vi "Camera Light.vi"(2 "Error In":errorcluster, 3 "input":dbl=250.0) -> (0 "Error Out":errorcluster)   [LabVIEW 2016]
doc: "This example demonstrates how to configure the SPI master and do a data loopback test using a LINX device."
uses:
  <vilib>/MakerHub/LINX/Private/Type Defs/Peripherals/SPI/SPI Configuration.ctl
  <vilib>/MakerHub/LINX/Private/Type Defs/Peripherals/SPI/SPI Bit Order.ctl
  <vilib>/MakerHub/LINX/Private/Type Defs/Peripherals/SPI/SPI Mode.ctl
  <vilib>/MakerHub/LINX/Public/Peripherals/SPI/SPI CS Config.ctl
  <vilib>/MakerHub/LINX/Private/Type Defs/Peripherals/SPI/SPI CS Logic Level.ctl
  <vilib>/MakerHub/LINX/Public/Peripherals/SPI/SPI Write Read 1 Frame.vi
  <vilib>/MakerHub/LINX/Public/Peripherals/SPI/SPI Write Read N Frames.vi
  <vilib>/MakerHub/LINX/Private/Local IO/LinxSpiWriteRead.vi
  <vilib>/MakerHub/LINX/Public/Utilities/Check Channel.vi
  <vilib>/MakerHub/LINX/Public/Utilities/Open Serial.vi
  <vilib>/MakerHub/LINX/Private/Utilties/Generate Error.vi
  <vilib>/MakerHub/LINX/LMH-LINX.lvlib
panel:
  in  "Data":u8[](array[numeric])=[24, 3]
  in  "Serial Port":refnum<visa-resource-name>="COM4"
  out "Read Data 2":u8[](array[numeric])
  out "Read Data":u8[](array[numeric])
  in  "CS Configuration":T1={"CS Channel"=10, "CS Logic Level"=enum."Active Low"}
  out "Actual Clock Frequency":u32
  in  "SPI Configuration":T3={"Clock Frequency"=1000000, "Bit Order"=enum."MSb First", "SPI Mode"=enum."Mode 1"}
  # "SPI Loop Back Example\n\nThis example demonstrates how to configure the SPI master and write one frame of SPI data.\n\nInstructions\n0. Connect (short) the SPI MOSI and MOSI pins.\n1. Select the COM Port associated with the LINX Device.\n2. Select the SPI Configuration.\n3. Select the CS Configuration.\n4. Click the Run Arrow.\n5. Enter some data in the Write Data control.  Notice the output on the Read Data indicator."
  # "Designer : Chin-Chia Kuo"
  # "INTT"
  # "LINX Device Settings"
  # "SPI Master Settings"
  # "SPI Write / Read Configruation"
  # "chip pick up tool 210"
  # "kapton tape : 50"
  # "sensor 15"
  # "please setting from 0 to 255"
  # "Recommend value \nSensor : 15\nDrill hole : 250"
  # "SPI Master Settings\n1. Set the target SPI clock frequency.  \n   The possible frequencies varies by device and the actual frequency used is returned.\n2. The bit order determines the order that the individual bits in each byte are shifted out.\n3. SPI Mode determines the clock polarity and phase. (View context help on the SPI Configure VI for more information)"
  # "SPI Write / Read Configuration\n1. Select the CS (chip select) DO channel.  The channel is automatically set as an output.\n2. Select the logic level for the CS pin.\n3. CS is automatically toggled each when the SPI Write / Read VI executes."
  # "SPI Write / Read Frame\n1. A 'frame' is one SPI transaction.  It starts when CS goes active and ends when CS returns to the idle state.\n2. A frame can be an arbitrary number for bytes in lenght.\n3. When using the SPI Write / Read VI in 1 Frame mode all data bytes are sent in a single frame.  For example if the data array contains 4 bytes all 4 bytes are sent as a single frame.\n4. When using the SPI Write / Read in N Frames mode the data bytes are divided into multiple frames.  \n    For example if the data array contains 4 bytes and the frame size is set to 2 the SPI Write / Read VI will send 2 frames of 2 bytes each.\n    The number of data bytes must be evenly divisble by the frame size."
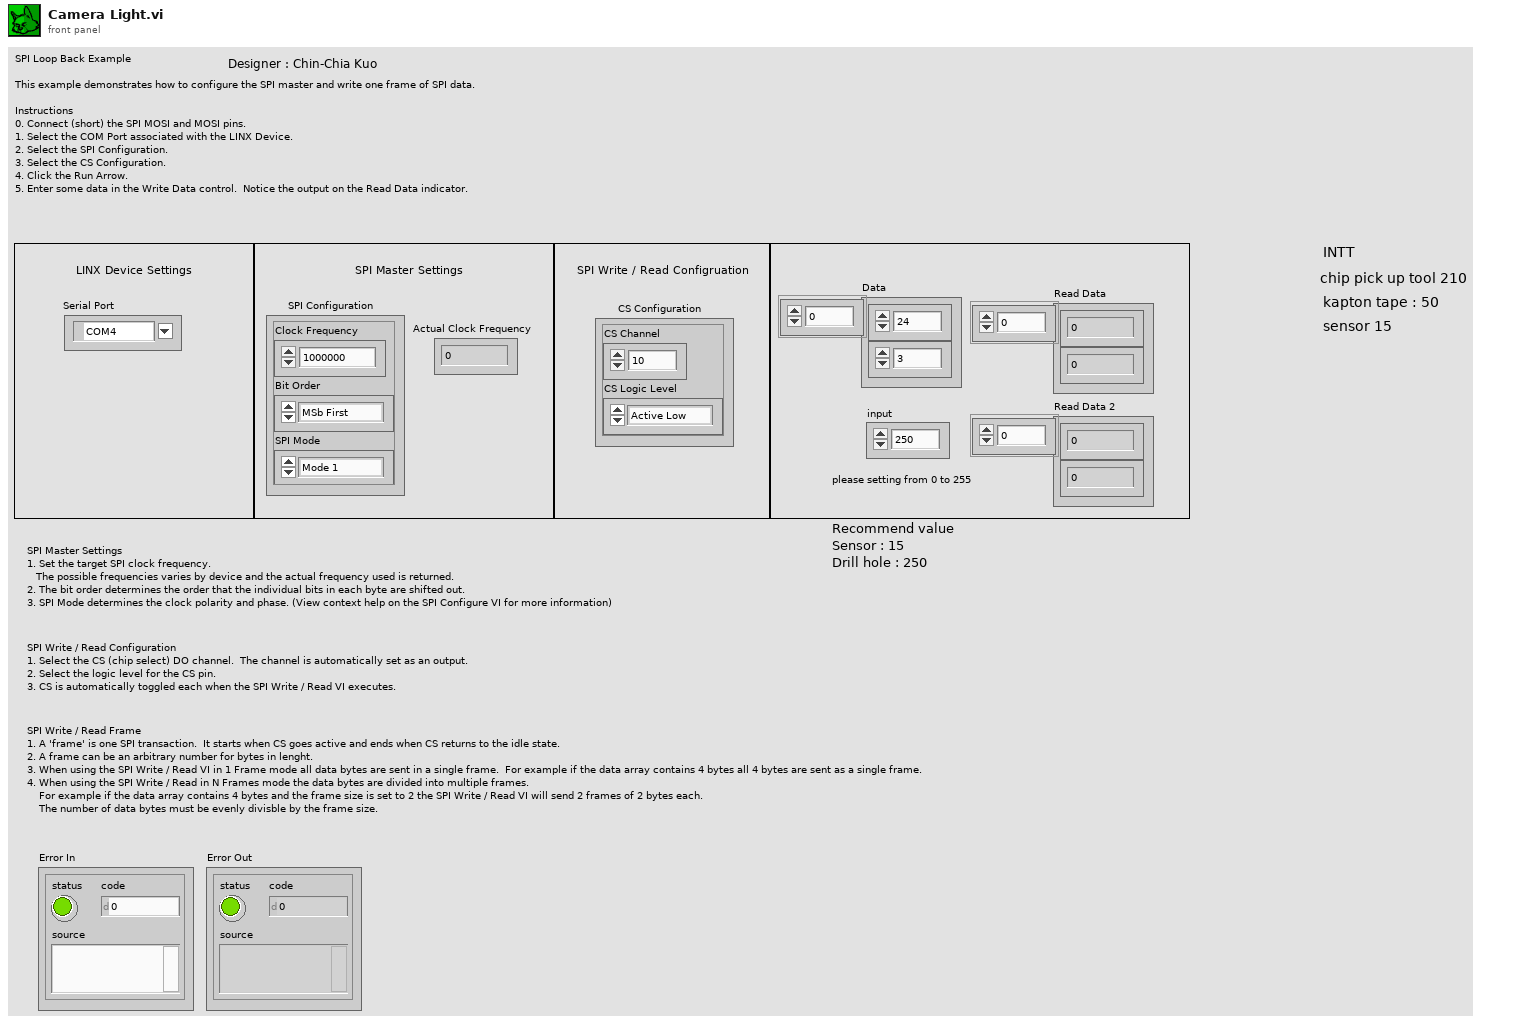
[diagram p1: front panel]
types:
  T1 = typedef "LMH-LINX.lvlib/SPI CS Config.ctl" = cluster{"CS Channel":u8, "CS Logic Level":T2}
  T2 = typedef "LMH-LINX.lvlib/SPI CS Logic Level.ctl" = enum8{"Active Low", "Active High"}
  T3 = typedef "LMH-LINX.lvlib/SPI Configuration.ctl" = cluster{"Clock Frequency":u32, "Bit Order":T4, "SPI Mode":T5}
  T4 = typedef "LMH-LINX.lvlib/SPI Bit Order.ctl" = enum8{"LSb First", "MSb First"}
  T5 = typedef "LMH-LINX.lvlib/SPI Mode.ctl" = enum8{"Mode 0", "Mode 1", "Mode 2", "Mode 3"}
  T6 = typedef "LMH-LINX.lvlib/LINX Ref.ctl" = cluster{"IO":T7, "Interface":T8, "LINX Device Config":T9}
  T7 = typedef "LMH-LINX.lvlib/Platform.ctl" = enum16{"Remote", "Local"}
  T8 = typedef "LMH-LINX.lvlib/Interface.ctl" = enum16{"Serial", "TCP"}
  T9 = typedef "LMH-LINX.lvlib/Device.lvlib/LINX Device Config.ctl" = cluster{"Interface":T8, "COM Port":refnum<visa-resource-name>, "TCP Configuration":T10, "Device Family":u8, "Device ID":u8, "Device Name":string, "TCP Ref":refnum<k5>, "Channels":T11}
  T10 = typedef "LMH-LINX.lvlib/Device.lvlib/TCP Config.ctl" = cluster{"IP Address":string, "Port":u16}
  T11 = typedef "LMH-LINX.lvlib/Channels.ctl" = cluster{"DI":u8[], "DO":u8[], "AI":u8[], "AO":u8[], "PWM":u8[], "QE":u8[], "UART":u8[], "I2C 2":u8[], "SPI":u8[], "CAN":u8[], "Servo":u8[], "AI Ref (V)":dbl, "AI Resolution (Bits)":u8, "AO Ref (V)":dbl, "AO Resolution (Bits)":u8}
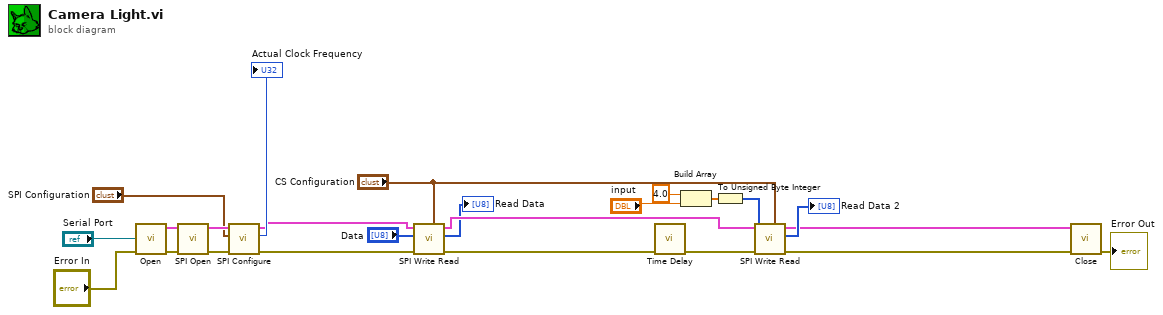
[diagram p0: block diagram]
diagram:
  n1 = call-poly <vilib>:"Open.vi"("Error In"="Error In", "Serial Port"="Serial Port") -> ("Error Out"=w21:errorcluster, "LINX Resource"=w24:T6)  [unwired: 7 in, 1 out]
  n2 = call <vilib>:"SPI Open.vi"("Error In"=w21, "LINX Resource"=w24) -> ("Error Out"=w22:errorcluster, "LINX Resource"=w23:T6)  [unwired: 8 in]
  n3 = call <vilib>:"SPI Configure.vi"("Error In"=w22, "SPI Configuration"="SPI Configuration", "LINX Resource"=w23) -> ("Error Out"=w3:errorcluster, "Actual Clock Frequency"=→"Actual Clock Frequency":u32, "LINX Resource"=w6:T6)  [unwired: 6 in]
  n4 = call-poly <vilib>:"SPI Write Read.vi"("CS Configuration"="CS Configuration", "Error In"=w3, "Data"="Data", "LINX Resource"=w6) -> ("Error Out"=w8:errorcluster, "Read Data"=→"Read Data":u8[], "LINX Resource"=w12:T6)  [unwired: 5 in]
  n5 = call "Time Delay"("error in (no error)"=w8) -> ("error out"=w11:errorcluster)  [unwired: 10 in]
  n6 = Build Array(4.0 ("element"), "input") -> (w15:dbl[])
  n7 = To Unsigned Byte Integer(number=w15) -> (unsigned 8bit integer=w17:u8[])
  n8 = call-poly <vilib>:"SPI Write Read.vi"("CS Configuration"="CS Configuration", "Error In"=w11, "Data"=w17, "LINX Resource"=w12) -> ("Error Out"=w4:errorcluster, "Read Data"=→"Read Data 2":u8[], "LINX Resource"=w5:T6)  [unwired: 5 in]
  n9 = call <vilib>:"Close.vi"("Error In"=w4, "LINX Resource"=w5) -> ("Error Out"=→"Error Out":errorcluster)  [unwired: 9 in]
